vi "4anumbersystem.vi"() -> ()   [LabVIEW 2013]
panel:
  out "Array":string[](array[string])
  in  "Ring":u16(ring) items=["Binary", "Octal", "Hexa"]
  in  "Input":dbl
  # "4a) Number System Conversion (Decimal to Other) using \n       case structure\n23A91A0459\nS.Nikhil Prince"
  # "MSB"
  # "LSB"
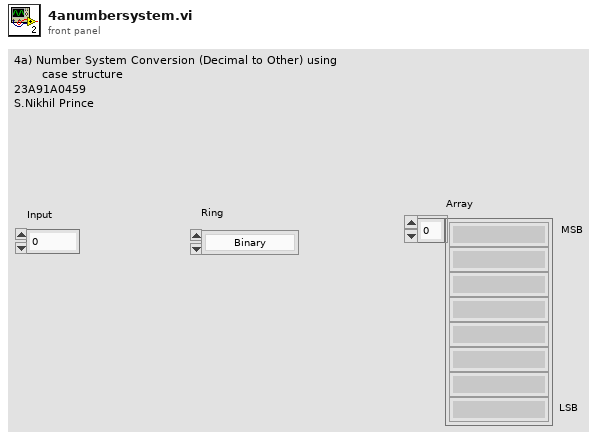
[diagram p1: front panel]
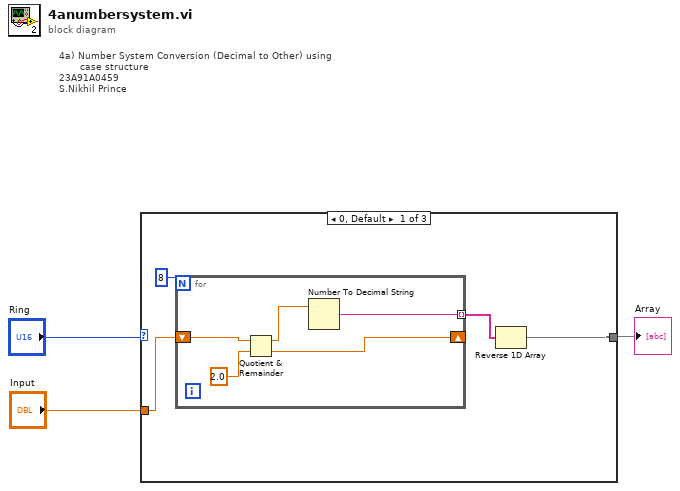
[diagram p0: block diagram]
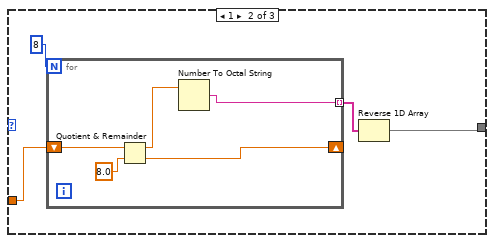
[diagram p2: hidden frame]
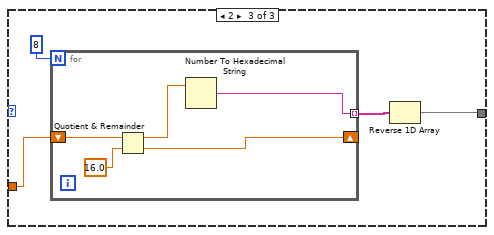
[diagram p3: hidden frame]
diagram:
  # "4a) Number System Conversion (Decimal to Other) using \n       case structure\n23A91A0459\nS.Nikhil Prince"
  n1 = case shown="0, Default" "Ring" {
    tunnel: "Input" -> [w6 w15 w24]
    tunnel: [w4 w14 w22] -> w1
    frame 0, Default {
      n2 = for {
        N: 8 -> [_]
        shift-right: [w9] -> _
        shift-left: w6 -> [w11]
        tunnel: [w8] -> w5 mode=indexing
        n3 = Quotient & Remainder(x=w11, y=2.0) -> (x-y*floor(x/y)=w10:dbl, floor(x/y)=w9:dbl)
        n4 = Number To Decimal String(number=w10) -> (decimal integer string=w8:string)  [unwired: 1 in]
      }
      n5 = Reverse 1D Array(array=w5) -> (reversed array=w4:string[])
    }
    frame 1 {
      n6 = for {
        N: 8 -> [_]
        shift-right: [w19] -> _
        shift-left: w15 -> [w20]
        tunnel: [w17] -> w13 mode=indexing
        n7 = Quotient & Remainder(x=w20, y=8.0 ("floor(x/y)")) -> (x-y*floor(x/y)=w18:dbl, floor(x/y)=w19:dbl)
        n8 = Number To Octal String(2:w18) -> (0:w17:string)  [unwired: 1 in]
      }
      n9 = Reverse 1D Array(array=w13) -> (reversed array=w14:string[])
    }
    frame 2 {
      n10 = for {
        N: 8 -> [_]
        shift-right: [w28] -> _
        shift-left: w24 -> [w29]
        tunnel: [w26] -> w23 mode=indexing
        n11 = Quotient & Remainder(x=w29, y=16.0) -> (x-y*floor(x/y)=w27:dbl, floor(x/y)=w28:dbl)
        n12 = Number To Hexadecimal String(2:w27) -> (0:w26:string)  [unwired: 1 in]
      }
      n13 = Reverse 1D Array(array=w23) -> (reversed array=w22:string[])
    }
  }
  "Array" <- w1
